vi "Agilent VNA Release.vi"(7 "Agilent VNA":T1, 8 "error in (no error)":errorcluster, 11 "VISA Resource Name":refnum<visa-resource-name>) -> (0 "error out":errorcluster {"code" format="%.0x"})   [LabVIEW 2011]
uses:
  TypeDefs/Agilent VNA Instrument Info.ctl
  TypeDefs/Agilent VNA Error Message Mode.ctl
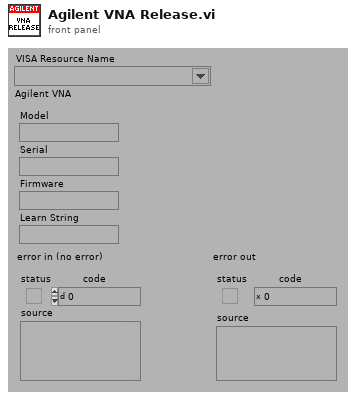
[diagram p1: front panel]
types:
  T1 = typedef "Agilent VNA Instrument Info.ctl" = cluster{"Model":string, "Serial":string, "Firmware":string, "Learn String":string}
  T2 = typedef "Agilent VNA Error Message Mode.ctl" = enum16{"On", "Off"}
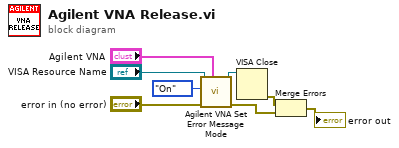
[diagram p0: block diagram]
diagram:
  n1 = call "Agilent VNA Set Error Message Mode.vi"("Agilent VNA"="Agilent VNA", "error in (no error)"="error in (no error)", "Error Message Mode"=Agilent_VNA_Error_Message_Mode."On", "VISA Resource Name"="VISA Resource Name") -> ("error out"=w4:errorcluster, "dup VISA Resource Name"=w1:refnum<visa-resource-name>)  [unwired: 6 out]
  n2 = VISA Close(VISA resource name=w1) -> (error out=w8:errorcluster)  [unwired: 1 in]
  n3 = Merge Errors(w8, w4) -> (→"error out":errorcluster)
